vi "Dashboard Main.vi"() -> ()   [LabVIEW 2013]
uses:
  <vilib>/Rock Robotics/WPI/Camera/WPI_CameraExposure Priority Values.ctl
  <vilib>/Rock Robotics/WPI/Camera/WPI_CameraWhite Balance Values.ctl
  <vilib>/Rock Robotics/WPI/Camera/WPI_CameraExposure Values.ctl
  <vilib>/Rock Robotics/WPI/Camera/WPI_CameraImageSize.ctl
  <vilib>/vision/Image Controls.llb/IMAQ Image.ctl
  <vilib>/Utility/error.llb/DialogType.ctl
  <vilib>/Utility/file.llb/Write To Spreadsheet File (string).vi
  <vilib>/addons/control/pid/pid.llb/PID Control Input Filter (DBL).vi
  <vilib>/vision/NI_Vision_Development_Module.lvlib
  <vilib>/addons/control/pid/NI_PID_pid.lvlib
  <vilib>/Analysis/NI_AALBase.lvlib
panel:
  in  "Cam File":enum32{"Auto Detect", "Sting", "Sister-Sting"}(radio)
  out "Person Change":bool
  out "standard deviation":dbl(knob) scale=0.0..1.0
  out "compass lag":dbl
  out "Frame Number":i32
  in  "Bank Shot":bool
  out "Status":T1(ring)
  out "Mode":enum8{"Tele-Op", "Auto", ""}(ring)=enum.""
  out "Ang":dbl(knob) scale=-10.0..10.0
  out "Dist":dbl(knob) scale=12.0..32.0
  out "Ball Count":dbl
  out "RIO Fire":bool
  in  "TargetMarginMin":dbl=5.0
  in  "TargetMarginMax":dbl=5.0
  in  "SteadyTimeLimit":dbl=1.0
  out "Processed Image 2":T2(plugin-control)
  out "Purple Settings":T3
  out "Red Settings":T3
  out "Blue Settings":T3
  out "Lum Range":cluster{i32, i32}
  out "Sat Range":cluster{i32, i32}
  out "Hue Range":cluster{i32, i32}
  out "SubFrame2":i32
  out "SubFrame1":i32
  out "Left Target Valid":bool
  out "Y2":dbl
  out "Right Target Valid":bool
  out "ScoreLowerLimitsA":dbl[](array[numeric])
  out "Processed Image Source":T2
  out "Scored Particle Info":T4(array[cluster])
  out "Scored Particle Info 2":T4(array[cluster])
  out "Processed Image 2 Source":T2
  out "Raw Image Out 2":T2
  out "Raw Image Out":T2
  out "Processed Image":T2(plugin-control)
  out "Right Target":T5
  out "Left Target":T5
  out "TargetAcquired":bool
  out "Rotated Image 2":T2(plugin-control)
  out "Rotated Image":T2(plugin-control)
  out "Softstops!":bool caption="FAILSAFE!"
  in  "Tab Control":T6(tab)
  out "Turrett SLOW Mode":bool
  out "Collector System Enabled":bool
  out "Shooter RPM":cluster{dbl, dbl}(knob)={0.0, 3890.9503656333954} scale=0.0..4000.0
  out "Limit Right":bool
  out "Limit Left":bool
  out "Turret Postition":cluster{dbl, dbl}(knob)={0.0, 3.981103692185485} scale=-240.0..60.0
  out "Home":bool
  out "1":bool
  out "2":bool
  out "3":bool
  out "Bridge Balance":bool
  out "Intake Direction":bool
  out "High Gear":bool
  out "Low Gear":bool
  out "Battery Voltage":dbl(slide) scale=8.0..14.0
  out "Distance From Target":dbl
  out "Angle to Target":dbl
  out "Entrance":bool
  out "Lower Belt":bool
  out "Upper Belt":bool
  out "Primed":bool
  out "AngleTolerance":dbl
  out "Auto Targeting":bool
  out "In Angle Range":bool
  out "Turret Enc":dbl
  out "Compass":dbl(knob) scale=0.0..-180.0
  out "Shooter Ready":bool
  out "Right Drive":dbl
  out "Left Drive":dbl
  out "Gyro":dbl(knob) scale=-180.0..180.0
  out "Robot IP Address":string
  out "In Angle?":bool
  out "Personality":string
  out "Cam File":string
  out "Lag":bool
  in  "Score Lower Limits":T7={"Rect Coverage"=76.0, "Aspect Ratio"=100.0, "X Edge Strength"=40.0, "Y Edge Strength"=60.0}
  in  "Aspect Ratio Upper":dbl=200.0
  in  "Distance Change":dbl
  in  "Left FOV":dbl=35.0
  in  "Right FOV":dbl=35.0
  in  "Area Size Limit":i32=444
  in  "Particle Count Limit":i32=8
  in  "Shift Right Camera  Right (Pixels)":dbl=-23.0
  in  "Shift Left Camera Right (Pixels)":dbl
  in  "Camera Width":dbl=18.0
  in  "Distance M Correction":dbl=1.3463
  in  "Distance B \nCorrection":dbl=2.0300000000000002
  out "Target Data":T8
  out "FPS":dbl
  in  "Angle Correction":dbl=1.0
  out "X1":dbl
  out "Y1":dbl
  out "X2":dbl
  in  "Color Level":i32(slide)=50 min=0 max=100 scale=0.0..100.0
  in  "Sharpness":i32(slide) min=0 max=100 scale=0.0..100.0
  in  "Brightness":i32(slide)=50 min=0 max=100 scale=0.0..100.0
  in  "Camera Settings":T10={"fps"=30, "compression"=30, "Image Size"=enum."640x480"}
  in  "Exposure Priority":T11=enum."Prioritize frame rate"
  in  "Exposure":T12=enum."Flicker-free 60 Hz"
  in  "White Balance":T13=enum."Fixed fluorescent 1"
  in  "Processed":bool
  in  "Sat":i32=255
  in  "Lum":i32=255
  in  "Hue":i32=40
  in  "Hue":i32(knob)=206 scale=0.0..255.0
  in  "Saturation":i32=80
  in  "Luminance":i32=20
  in  "LED Colors":enum16{"Blue", "Red", "Purple", "Test"}(ring)=enum."Purple"
  in  "Reload":bool
  in  "Write Blue":bool
  in  "Write Red":bool
  in  "Write Purple":bool
  in  "Calibrate Cameras":bool
  in  "Distance to Target":dbl=16.8
  out "FIRE!":bool
  out "Dashboard Datatype Warning":string="Warning: The Dashboard Datatype used by the robot project and this dashboard do not match.\nSee diagram for more details."
  # "The different autonomous can be set up from the driver station. Set up as binary.\n1 (001) - Default\n2 (010)- Coopertition (have another bot feed us balls that we can shoot, untested)\n3 (011)- X second delay to shooting first ball (NO BRIDGE)\n4 (100) - X second delay to shooting first ball (Go for bridge)\n5 (101)- Reverse Order (Puts down bridge then shoots, untested)"
  # "Ball Count"
  # "Communications"
  # "Margin"
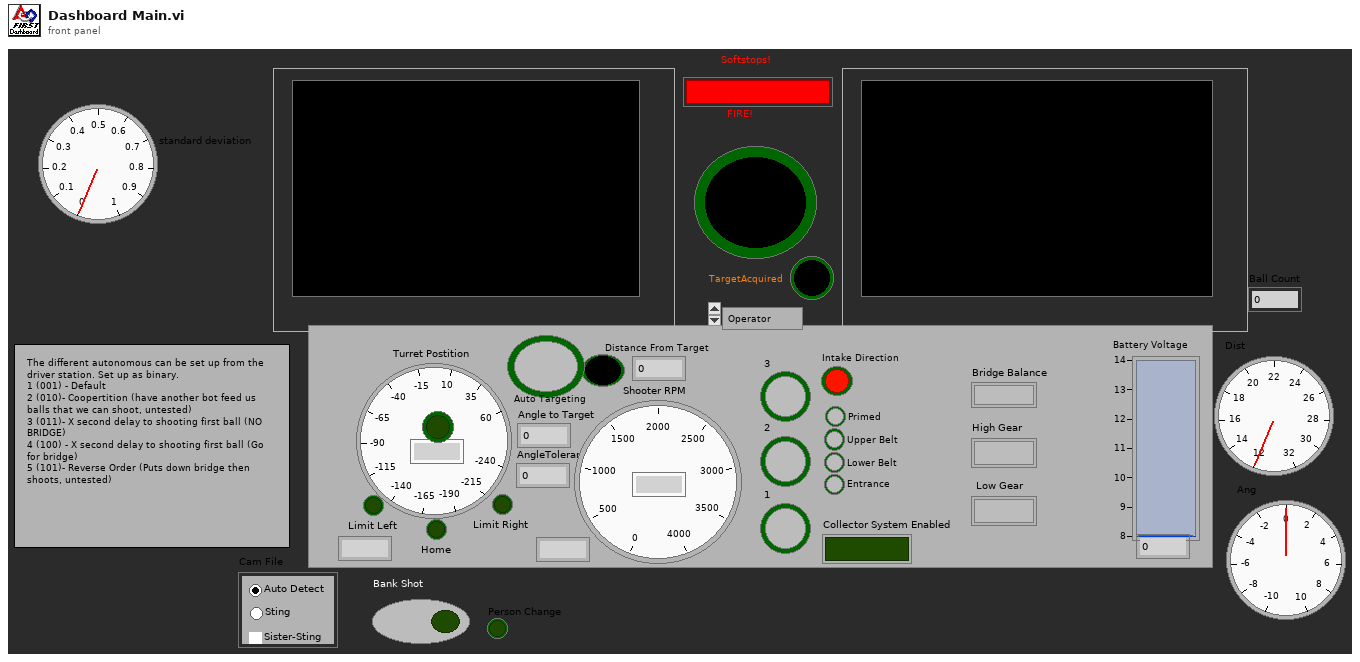
[diagram p1: front panel]
types:
  T1 = enum8{"Disconnected", "E-Stop", "Disabled", "Enabled"}
  T2 = typedef "IMAQ Image.ctl" = refnum<image>
  T3 = cluster{cluster{"Hue":i32, "Sat":i32, "Lum":i32}, cluster{"HueM":i32, "SatM":i32, "LumM":i32}}
  T4 = cluster{cluster{"Left":dbl, "Top":dbl, "Right":dbl, "Bottom":dbl}, dbl[]}[]
  T5 = cluster{"Left":dbl, "Top":dbl, "Right":dbl, "Bottom":dbl}
  T6 = enum32{"Operator", "Diagnotics", "Vision", "Camera Conf"}
  T7 = cluster{"Rect Coverage":dbl, "Aspect Ratio":dbl, "X Edge Strength":dbl, "Y Edge Strength":dbl}
  T8 = cluster{i32, dbl, "Angle to Target":dbl, "Valid Target":bool}
  T9 = typedef "WPI_CameraImageSize.ctl" = enum16{"640x480", "320x240", "160x120"}
  T10 = cluster{"fps":i32, "compression":i32, "Image Size":T9}
  T11 = typedef "WPI_CameraExposure Priority Values.ctl" = enum16{"None", "Prioritize frame rate", "Prioritize image quality"}
  T12 = typedef "WPI_CameraExposure Values.ctl" = enum16{"Auto", "Flicker-free 50 Hz", "Flicker-free 60 Hz", "Hold current"}
  T13 = typedef "WPI_CameraWhite Balance Values.ctl" = enum16{"Auto", "Fixed indoor", "Fixed outdoor 1", "Fixed outdoor 2", "Fixed fluorescent 1", "Fixed fluorescent 2", "Hold current"}
  T14 = cluster{"Bridge Balance":bool, "Gyro":dbl, "Left Drive":dbl, "Right Drive":dbl, "Shooter Ready":bool, "Compass":dbl, "Turret Enc":dbl, "Gear":u16, "Turret Postion":dbl, "Turret Bump":bool, "Collector System Enabled?":bool, "Personality":string}
  T15 = cluster{"Ball Count":dbl, "Shooter RMP":dbl, "FIRE":bool, "FailSafe":bool, "Entrance":bool, "Lower Belt":bool, "Upper Belt":bool, "Primed":bool, "Intake":bool, "Right Limit":bool, "Home":bool, "Left Limit":bool, "Auto Target ?":bool}
  T16 = typedef "Image Type" = u32
  T17 = typedef "DialogType.ctl" = u16
  T18 = cluster{"Competition mode":bool, "Robot Link":bool, "Autonomous":bool, "Enabled":bool, "E-Stop":bool}
  T19 = cluster{"Distance From Target":dbl, "Distance From Target":dbl, "Distance From Target":dbl, "Distance From Target":dbl, "Distance From Target":dbl}
  T20 = cluster{"Shooter RMP":dbl, "Shooter RPM Control":dbl}
  T21 = typedef "WPI_CameraDevRef.ctl" = cluster{"Camera Address":string, "CameraStatus":errorcluster, "Acquire Image Notifier":refnum<notifier>}
  T22 = typedef "LVRectTypeDef.ctl" = cluster{"Left":i16, "Top":i16, "Right":i16, "Bottom":i16}
  T23 = cluster{"SteadyTime":dbl, "TargetMarMax":dbl, "TargetMarMin":dbl}
  T24 = cluster{cluster{"LFOV":dbl, "RFOV":dbl, "CamW":dbl}, cluster{"Ladj":dbl, "Radj":dbl, "Dadj":dbl}, cluster{"CamM":dbl, "CamB":dbl, "AngM":dbl}, "Color":u16}
  T25 = cluster{"Hue":i32, "Saturation":i32, "Luminance":i32}
  T26 = cluster{cluster{"Hue":i32, "Saturation":i32, "Luminance":i32}, cluster{"Hue":i32, "Sat":i32, "Lum":i32}}
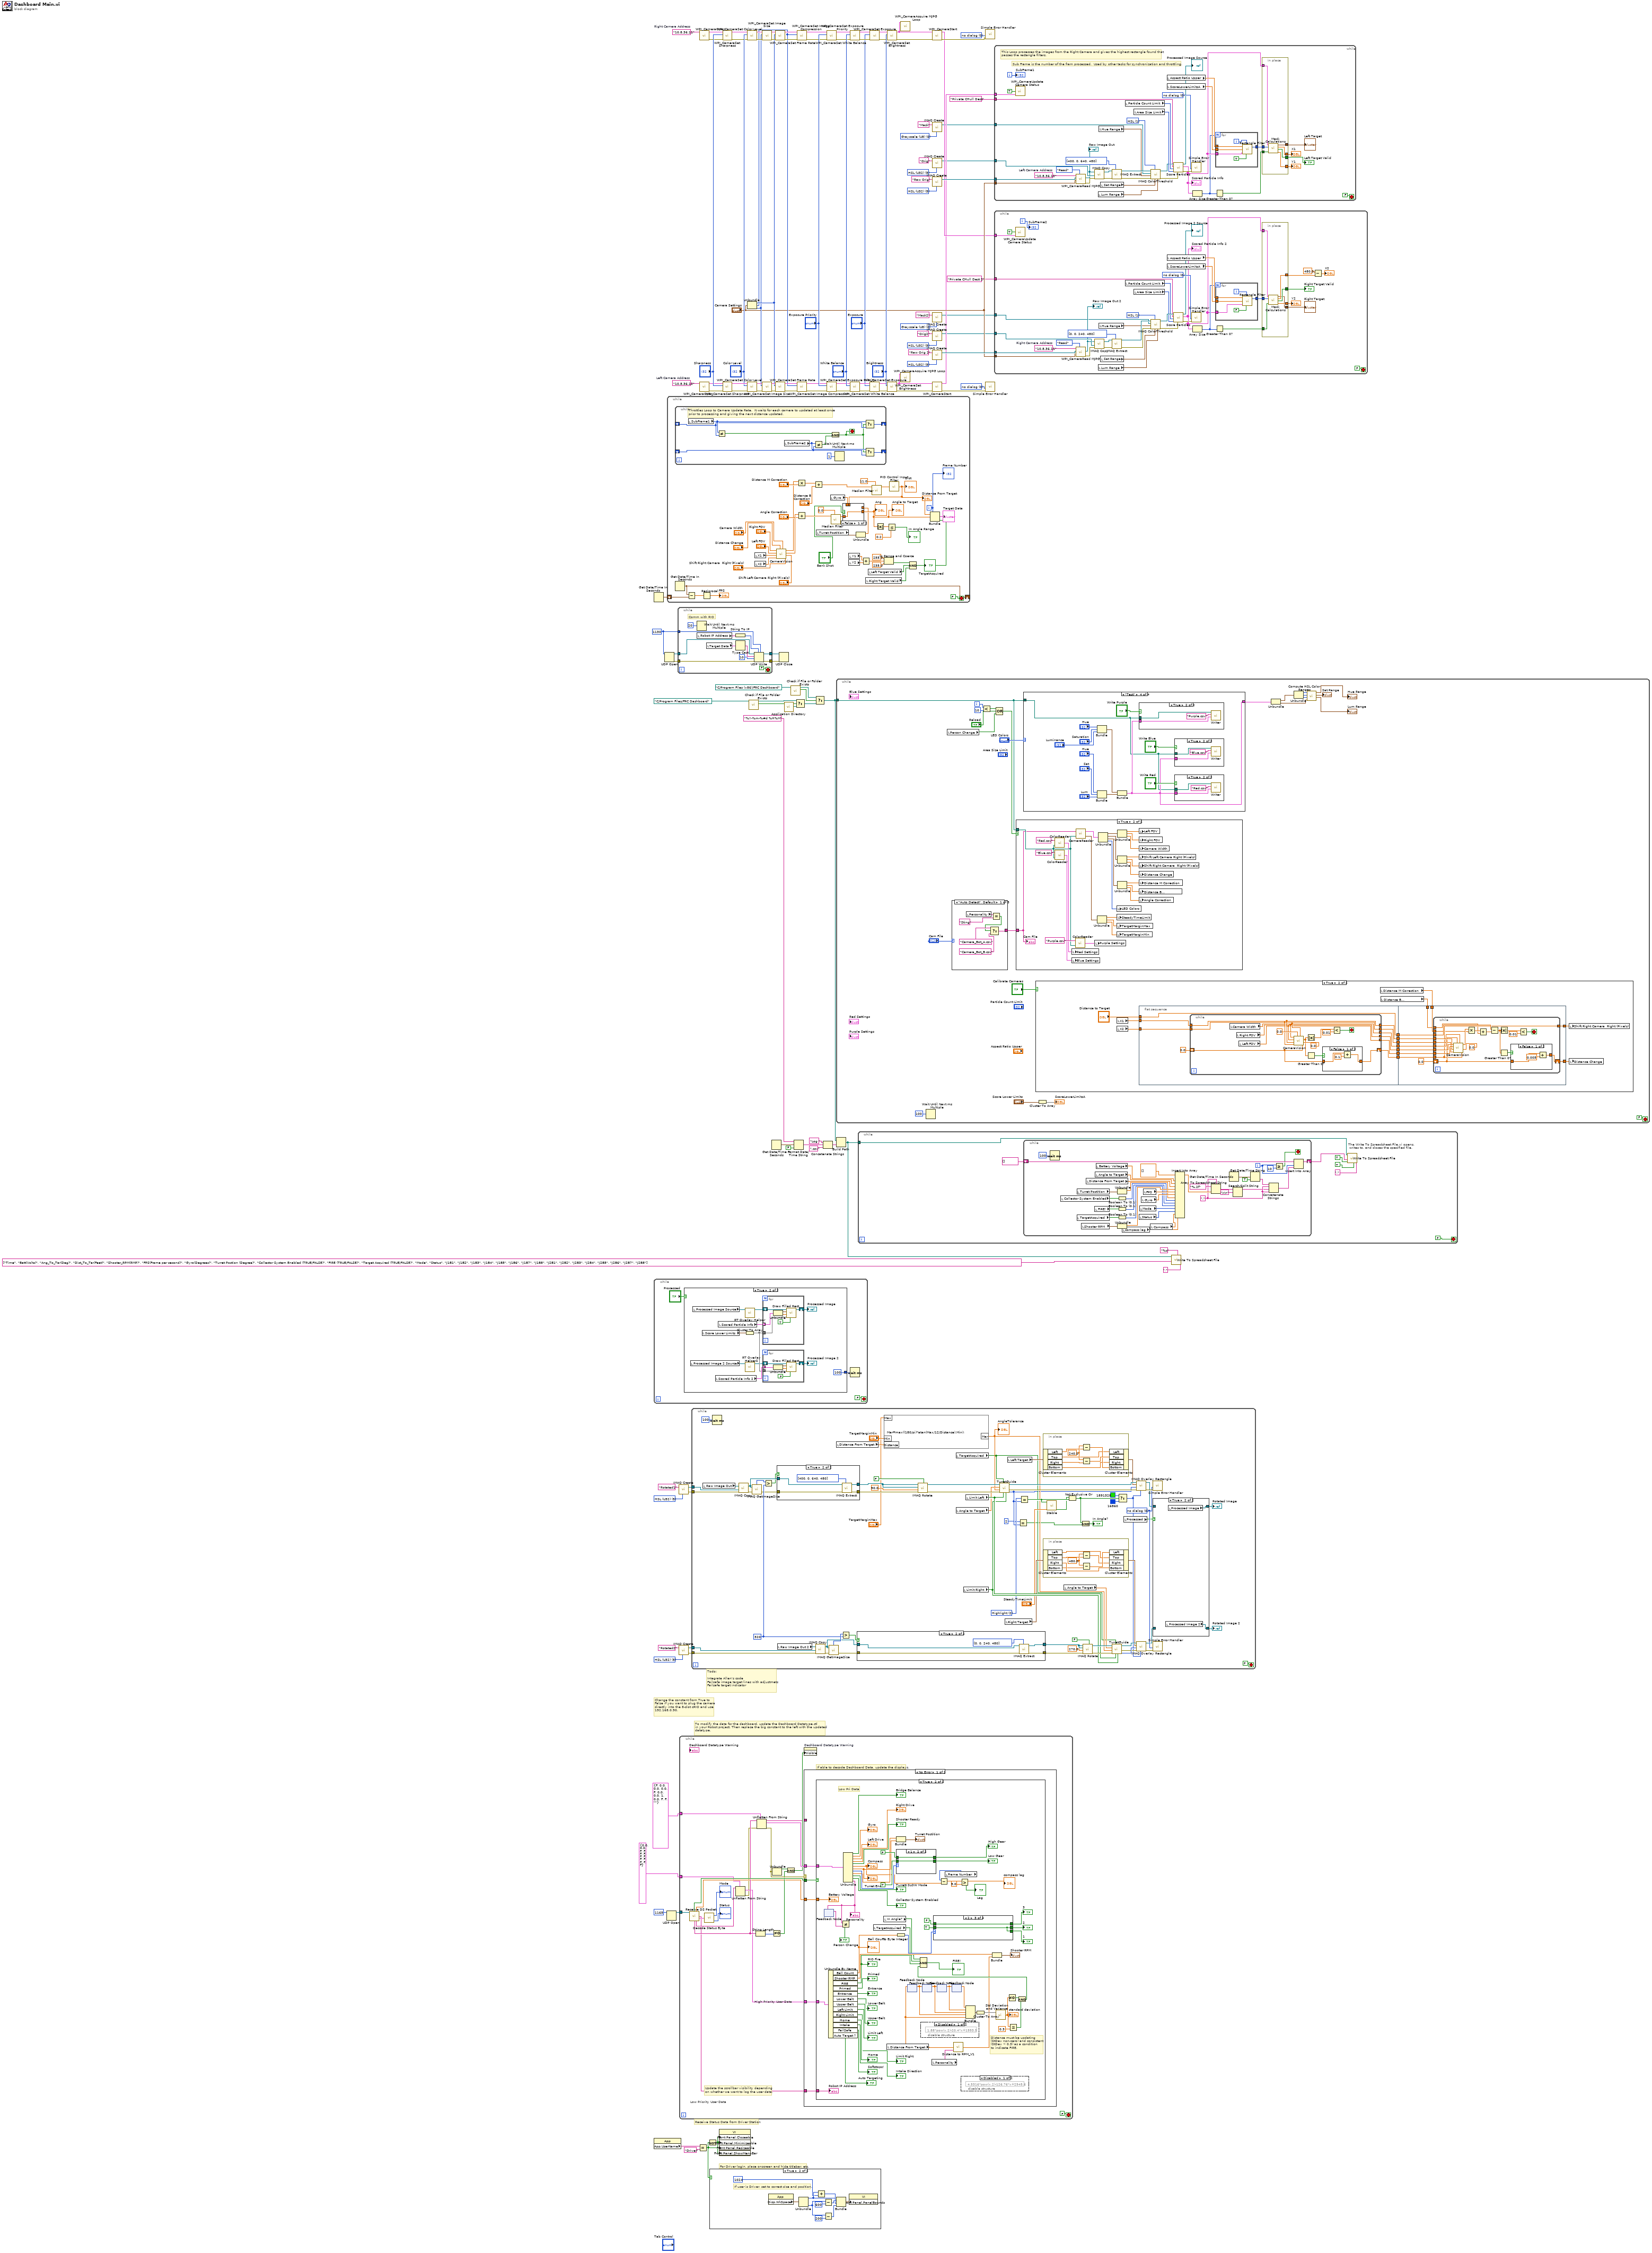
[diagram p0: block diagram]
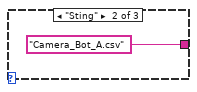
[diagram p2: hidden frame]
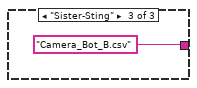
[diagram p3: hidden frame]
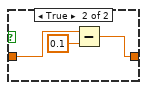
[diagram p5: hidden frame]
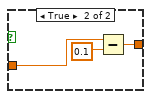
[diagram p6: hidden frame]
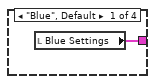
[diagram p8: hidden frame]
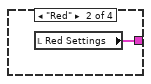
[diagram p9: hidden frame]
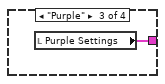
[diagram p10: hidden frame]
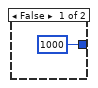
[diagram p14: hidden frame]
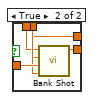
[diagram p19: hidden frame]
diagram:
  w7 = T16 5 items=["Grayscale (U8)", "Grayscale (I16)", "Grayscale (SGL)", "Complex (CSG)", "RGB (U32)", "HSL (U32)", "RGB (U64)", "Grayscale (U16)"] ("Image Type")
  w9 = T16 0 items=["Grayscale (U8)", "Grayscale (I16)", "Grayscale (SGL)", "Complex (CSG)", "RGB (U32)", "HSL (U32)", "RGB (U64)", "Grayscale (U16)"] ("Image Type")
  w12 = T16 0 items=["Grayscale (U8)", "Grayscale (I16)", "Grayscale (SGL)", "Complex (CSG)", "RGB (U32)", "HSL (U32)", "RGB (U64)", "Grayscale (U16)"] ("Image Type")
  w16 = T16 5 items=["Grayscale (U8)", "Grayscale (I16)", "Grayscale (SGL)", "Complex (CSG)", "RGB (U32)", "HSL (U32)", "RGB (U64)", "Grayscale (U16)"] ("Image Type")
  w21 = T17 0 items=["no dialog", "OK message", "continue or stop message", "OK message + warnings", "continue/stop + warnings"] ("type of dialog (OK msg:1)")
  w22 = T17 0 items=["no dialog", "OK message", "continue or stop message", "OK message + warnings", "continue/stop + warnings"] ("type of dialog (OK msg:1)")
  w28 = T16 5 items=["Grayscale (U8)", "Grayscale (I16)", "Grayscale (SGL)", "Complex (CSG)", "RGB (U32)", "HSL (U32)", "RGB (U64)", "Grayscale (U16)"] ("Image Type")
  w30 = T16 5 items=["Grayscale (U8)", "Grayscale (I16)", "Grayscale (SGL)", "Complex (CSG)", "RGB (U32)", "HSL (U32)", "RGB (U64)", "Grayscale (U16)"] ("Image Type")
  w26 = "10.8.36.11"  # Right Camera Address
  w32 = "10.8.36.12"  # Left Camera Address
  w107 = T16 5 items=["Grayscale (U8)", "Grayscale (I16)", "Grayscale (SGL)", "Complex (CSG)", "RGB (U32)", "HSL (U32)", "RGB (U64)", "Grayscale (U16)"] ("Image Type")
  w110 = T16 5 items=["Grayscale (U8)", "Grayscale (I16)", "Grayscale (SGL)", "Complex (CSG)", "RGB (U32)", "HSL (U32)", "RGB (U64)", "Grayscale (U16)"] ("Image Type")
  w111 = u16 1130 ("port")
  # "Todo: \n\nIntegrate Allen's code\nFailsafe image target lines with adjustmets\nFailsafe target indicator"
  # "Change the constant from True to\nFalse if you want to plug the camera\ndirectly into the 8-slot cRIO and use\n192.168.0.90."
  # "For Driver login, place onscreen and hide titlebar, etc."
  # "To modify the data for the dashboard, update the Dashboard Datatype.ctl\nin your Robot project. Then replace the big constant to the left with the updated\ndatatype."
  # "Receive Status Data from Driver Station"
  n1 = Get Date/Time In Seconds() -> (seconds since 1Jan1904=w116:timestamp)
  n2 = while {
    stop <- FALSE stop-if-true
    n3 = case shown="True" "Processed" {
      tunnel: [u32 1000 ("milliseconds to wait") u32 100 ("milliseconds to wait")] -> w121
      frame False {
      }
      frame True {
        n4 = local read "Processed Image 2 Source"() -> (w134:T2)
        n5 = local read "Processed Image Source"() -> (w131:T2)
        n6 = local read "Score Lower Limits"() -> (w135:T7)
        n7 = local read "Scored Particle Info 2"() -> (w133:T4)
        n8 = local read "Scored Particle Info"() -> (w130:T4)
        n9 = call "RT Overlay Helper.vi"("Refnum in"=w131) -> ("Refnum out"=w126:T2)  [unwired: 10 in]
        n10 = Cluster To Array(cluster=w135) -> (array=w132:dbl[])
        n11 = call "RT Overlay Helper2.vi"("Refnum in"=w134) -> ("Refnum out"=w128:T2)  [unwired: 10 in]
        n12 = for {
          shift-right: [w141] -> w127
          shift-left: w126 -> [w142]
          tunnel: w130 -> [w138] mode=indexing
          tunnel: w132 -> [w137]
          n13 = Unbundle(w138) -> (w139:T5, w140:dbl[])
          n14 = call "Draw Filled Rect.vi"("Left"=TRUE, "Limits"=w137, "Scores"=w140, "Bounding Box"=w139, "image in"=w142) -> ("image out"=w141:T2)  [unwired: 6 in]
        }
        "Processed Image" <- w127
        n15 = for {
          shift-right: [w148] -> w129
          shift-left: w128 -> [w149]
          tunnel: w133 -> [w145] mode=indexing
          tunnel: w132 -> [w144]
          n16 = Unbundle(w145) -> (w146:T5, w147:dbl[])
          n17 = call "Draw Filled Rect.vi"("Left"=FALSE, "Limits"=w144, "Scores"=w147, "Bounding Box"=w146, "image in"=w149) -> ("image out"=w148:T2)  [unwired: 6 in]
        }
        "Processed Image 2" <- w129
      }
    }
    n18 = Wait (ms)(milliseconds to wait=w121) -> ()  [unwired: 1 out]
  }
  n19 = property class="App"() -> ("App.UserName"=w117:string)  [unwired: 2 in, 2 out]
  n20 = UDP Open(11:w111) -> (port=w114:refnum<k16>, 0:w112:errorcluster)  [unwired: 4 in, 1 out]
  n21 = UDP Open(11:u16 1165 ("port")) -> (port=w119:refnum<k16>)  [unwired: 2 in, 4 out]
  n22 = while {
    shift-right: [w168] -> _
    shift-left: w116 -> [w190]
    i -> [w182]
    stop <- FALSE stop-if-true
    n23 = while {
      shift-right: [w209] -> _
      shift-left: _ -> [w207]
      shift-right: [w206] -> _
      shift-left: _ -> [w205]
      stop <- w201 stop-if-true
      # "Throttles Loop to Camera Update Rate.  It waits for each camera to updated at least once\nprior to processing and giving the next distance updated."
      n24 = local read "SubFrame1"() -> (w208:i32)
      n25 = Not Equal?(x=w208, y=w207) -> (x != y?=w202:bool)
      n26 = local read "SubFrame2"() -> (w204:i32)
      n27 = Not Equal?(x=w204, y=w205) -> (x != y?=w203:bool)
      n28 = And(x=w202, y=w203) -> (x .and. y?=w201:bool)
      n29 = Wait Until Next ms Multiple(millisecond multiple=u32 1) -> ()  [unwired: 1 out]
      n30 = Select(t=w208, s=w201, f=w207) -> (s? t:f=w209:i32)
      n31 = Select(t=w204, s=w201, f=w205) -> (s? t:f=w206:i32)
    }
    n32 = Get Date/Time In Seconds() -> (seconds since 1Jan1904=w168:timestamp)
    n33 = Subtract(x=w168, y=w190) -> (x-y=w165:dbl)
    n34 = Reciprocal(x=w165) -> (1/x=→"FPS":dbl)
    n35 = local read "X1"() -> (w170:dbl)
    n36 = local read "X2"() -> (w174:dbl)
    n37 = call "CameraVision.vi"("X2 Change"="Shift Right Camera  Right (Pixels)", "X1 Change"="Shift Left Camera Right (Pixels)", "W"="Camera Width", "Distance Change"="Distance Change", "x2"=w174, "x"=w170, "Left FOV"="Left FOV", "Right FOV"="Right FOV") -> ("Angle to Target"=w184:dbl, "Distance to Target"=w181:dbl)  [unwired: 1 in]
    n38 = Multiply(x=w181, y="Distance M Correction") -> (x*y=w176:dbl)
    n39 = Add(x=w184, y="Angle Correction") -> (x+y=w163:dbl)
    n40 = Add(x=w176, y="Distance B \nCorrection") -> (x+y=w162:dbl)
    n41 = local read "Turret Postition"() -> (w154:cluster{dbl, dbl})
    n42 = local read "Gyro"() -> (w152:dbl)
    n43 = call "Median Filter.vi"("Initial Value"=0.0, "Variable"=w163) -> ("Filtered Value"=w156:dbl)  [unwired: 9 in]
    n44 = local read "Y1"() -> (w169:dbl)
    n45 = local read "Y2"() -> (w172:dbl)
    n46 = Unbundle(w154) -> (w153:dbl)  [unwired: 1 out]
    n47 = Add(x=w169, y=w172) -> (x+y=w179:dbl)
    n48 = local read "Right Target Valid"() -> (w173:bool)
    n49 = local read "Left Target Valid"() -> (w171:bool)
    n50 = call "Median Filter.vi"("Initial Value"=11.0, "Variable"=w162) -> ("Filtered Value"=w161:dbl)  [unwired: 9 in]
    n51 = In Range and Coerce(upper limit=255.0, x=w179, lower limit=235.0) -> (In Range?=w150:bool)  [unwired: 1 out]
    n52 = call-poly <vilib>:"PID Control Input Filter.vi"("input"=w161) -> ("output"=w155:dbl)  [unwired: 4 in]
    "Distance From Target" <- w155
    "Dist" <- w155
    n53 = case shown="False" "Bank Shot" {
      tunnel: [w195 w200] -> w157
      tunnel: w156 -> [w195 w199]
      tunnel: w155 -> [_ w198]
      tunnel: w153 -> [_ w197]
      tunnel: w152 -> [_ w196]
      frame False {
      }
      frame True {
        n54 = call "Bank Shot.vi"("L (ft)"=w198, "Camera (deg)"=w199, "Turret (deg)"=w197, "Gryo (deg)"=w196) -> ("C Prime"=w200:dbl)  [unwired: 6 in, 1 out]
      }
    }
    "Angle to Target" <- w157
    "Ang" <- w157
    n55 = Absolute Value(x=w157) -> (abs(x)=w160:dbl)
    n56 = Less Or Equal?(x=w160, y=0.2) -> (x <= y?=→"In Angle Range":bool)
    n57 = Compound Arithmetic op=AND(w150, w171, w173) -> (w175:bool)
    "TargetAcquired" <- w175
    n58 = Bundle(w182, "output"=w155, "C Prime"=w157, w175) -> (→"Target Data":cluster{i32, "output":dbl, "C Prime":dbl, bool})  [unwired: 1 in]
    "Frame Number" <- w182
  }
  n59 = while {
    tunnel: [w217] -> w115
    tunnel: w114 -> [w216]
    tunnel: [w218] -> w113
    tunnel: w112 -> [w213]
    tunnel: w111 -> [w212]
    stop <- FALSE stop-if-true
    # "Comm with RIO"
    n60 = Wait Until Next ms Multiple(millisecond multiple=u32 20) -> ()  [unwired: 1 out]
    n61 = local read "Robot IP Address"() -> (w211:string)
    n62 = local read "Target Data"() -> (w219:T8)
    n63 = String To IP(1:w211) -> (0:w220:u32)
    n64 = Type Cast(x=w219) -> (*(type *) &x=w215:string)  [unwired: 1 in]
    n65 = UDP Write(address=w220, port or service name=w212, connection ID=w216, data in=w215, 8:w213, 9:10 ("timeout ms (25000)")) -> (error out=w218:errorcluster, 3:w217:refnum<k16>)
  }
  n66 = call "IMAQ Create"("Image Name"="Rotated1", "Image Type"=w110) -> ("New Image"=w106:T2, "error out"=w103:errorcluster)  [unwired: 2 in, 1 out]
  n67 = call "IMAQ Create"("Image Name"="Rotated2", "Image Type"=w107) -> ("New Image"=w105:T2, "error out"=w104:errorcluster)  [unwired: 2 in, 1 out]
  n68 = while {
    tunnel: w119 -> [w241]
    tunnel: T14 {"Bridge Balance"=FALSE, "Gyro"=0.0, "Left Drive"=0.0, "Right Drive"=0.0, "Shooter Ready"=FALSE, "Compass"=0.0, "Turret Enc"=0.0, "Gear"=1, "Turret Postion"=0.0, "Turret Bump"=FALSE, "Collector System Enabled?"=FALSE, "Personality"=""} ("Dashboard Data") -> [w240]
    tunnel: T15 {"Ball Count"=0.0, "Shooter RMP"=0.0, "FIRE"=FALSE, "FailSafe"=FALSE, "Entrance"=FALSE, "Lower Belt"=FALSE, "Upper Belt"=FALSE, "Primed"=FALSE, "Intake"=FALSE, "Right Limit"=FALSE, "Home"=FALSE, "Left Limit"=FALSE, "Auto Target ?"=FALSE} ("HiPri") -> [w227]
    stop <- FALSE stop-if-true
    # "High Priority User Data"
    # "Low Priority User Data"
    # "Update the scrollbar visibility depending\non whether we want to log the user data."
    # "If able to decode Dashboard Data, update the displays."
    n69 = call "Receive DS Packet.vi"("Recv Socket"=w241) -> ("New Dashboard Data"=w237:bool, "Battery"=w229:sgl, "Robot IP Address"=w228:string, "Status"=w242:T18, "Low Priority User Data"=w231:string, "High Priority User Data"=w230:string)  [unwired: 1 in, 8 out]
    n70 = call "Decode Status Byte.vi"("Status Byte"=w242) -> ("Mode"=→"Mode":enum8{"Tele-Op", "Auto", ""}, "Status"=→"Status":T1)
    n71 = Unflatten From String(type=w227, binary string=w230) -> (value=w226:T15, error out=w225:errorcluster)  [unwired: 1 in, 3 out]
    n72 = String Length(string=w231) -> (length=w232:i32)
    n73 = Unflatten From String(type=w240, binary string=w231, error in (no error)=w225) -> (rest of the binary string=w233:string, value=w239:T14, error out=w238:errorcluster)  [unwired: 2 out]
    n74 = Not Equal To 0?(x=w232) -> (x != 0?=w235:bool)
    n75 = Unbundle(w238) -> ("status"=w234:bool)  [unwired: 2 out]
    n76 = And(x=w234, y=w235) -> (x .and. y?=w236:bool)
    n77 = property on="Dashboard Datatype Warning" class="Str"("Visible"=w236) -> ()  [unwired: 2 in, 2 out]
    n78 = case shown="No Error" w238 {
      tunnel: w239 -> [w248 _]
      tunnel: w237 -> [w247 _]
      tunnel: w233 -> [_ _]
      tunnel: w229 -> [w246 _]
      tunnel: w228 -> [w245 _]
      tunnel: w226 -> [w244 _]
      frame No Error {
        n79 = case shown="True" w247 {
          tunnel: w248 -> [_ w312]
          tunnel: w246 -> [_ w311]
          tunnel: w245 -> [_ w310]
          tunnel: w244 -> [_ w309]
          frame False {
            # "Don't update if the robot hasn't sent new data"
          }
          frame True {
            # "Distance must be updating\n(StDev non-zero) and consistent\n(StDev < 0.3) as a condition\nto indicate FIRE."
            # "Low Pri Data"
            n80 = feedback #1() -> (w250:string)  [unwired: 1 in]
            n81 = Unbundle By Name(w309) -> ("Ball Count"=w273:dbl, "Shooter RMP"=w282:dbl, "FIRE"=w276:bool, "Primed"=→"Primed":bool, "Entrance"=→"Entrance":bool, "Lower Belt"=→"Lower Belt":bool, "Upper Belt"=→"Upper Belt":bool, "Left Limit"=→"Limit Left":bool, "Right Limit"=→"Limit Right":bool, "Home"=→"Home":bool, "Intake"=→"Intake Direction":bool, "FailSafe"=→"Softstops!":bool, "Auto Target ?"=→"Auto Targeting":bool)
            "RIO Fire" <- w276
            "Ball Count" <- w273
            n82 = Unbundle(w312) -> ("Bridge Balance"=→"Bridge Balance":bool, "Gyro"=→"Gyro":dbl, "Left Drive"=→"Left Drive":dbl, "Right Drive"=→"Right Drive":dbl, "Shooter Ready"=→"Shooter Ready":bool, "Compass"=w271:dbl, "Turret Enc"=w275:dbl, "Gear"=w308:u16, "Turret Postion"=w280:dbl, "Turret Bump"=→"Turrett SLOW Mode":bool, "Collector System Enabled?"=→"Collector System Enabled":bool, "Personality"=w251:string)
            "Compass" <- w271
            "Turret Enc" <- w275
            "Personality" <- w251
            n83 = feedback-in #1(w251) -> ()
            n84 = Not Equal?(x=w251, y=w250) -> (x != y?=→"Person Change":bool)
            n85 = local read "TargetAcquired"() -> (w274:bool)
            n86 = local read "In Angle?"() -> (w277:bool)
            n87 = local read "Distance From Target"() -> (w254:dbl)
            n88 = Bundle("Turret Postion"=w280, "Turret Enc"=w275) -> (→"Turret Postition":cluster{"Turret Postion":dbl, "Turret Enc":dbl})  [unwired: 1 in]
            n89 = case shown="1" w308 {
              tunnel: [w320 w322] -> w307
              tunnel: FALSE -> [w319 w322]
              tunnel: TRUE -> [w320 w321]
              tunnel: [w319 w321] -> w304
              frame 0, Default {
              }
              frame 1 {
              }
            }
            "Low Gear" <- w304
            "High Gear" <- w307
            n90 = To Byte Integer(number=w273) -> (8bit integer=w289:i8)
            n91 = feedback-in #2(w254) -> ()
            n92 = feedback #2() -> (w262:dbl)  [unwired: 1 in]
            n93 = disable-structure shown="Disabled" {
              frame Disabled {
                n94 = expression code="1.88*pow(x,2)-20.4*x+1993.5"() -> ()  [unwired: 1 in, 1 out]
              }
              frame Enabled {
              }
            }
            n95 = feedback #3() -> (w263:dbl)  [unwired: 1 in]
            n96 = feedback-in #3(w262) -> ()
            n97 = local read "Personality"() -> (w252:string)
            n98 = case shown="2" w289 {
              tunnel: [w313 w314 w316 w318] -> w288
              tunnel: [w313 w314 w317 w318] -> w287
              tunnel: [w313 w315 w317 w318] -> w286
              tunnel: FALSE -> [w313 w314 w316 _]
              tunnel: TRUE -> [_ w315 w317 w318]
              frame 0, Default {
              }
              frame 1 {
              }
              frame 2 {
              }
              frame 3 {
              }
            }
            "3" <- w288
            "2" <- w287
            "1" <- w286
            n99 = feedback #4() -> (w264:dbl)  [unwired: 1 in]
            n100 = feedback-in #4(w263) -> ()
            n101 = local read "Frame Number"() -> (w270:i32)
            n102 = Subtract(x=w270, y=w271) -> (x-y=w269:dbl)
            "compass lag" <- w269
            n103 = feedback #5() -> (w265:dbl)  [unwired: 1 in]
            n104 = feedback-in #5(w264) -> ()
            n105 = call "Distance to RPM_V1.vi"("Personality"=w252, "Target Distance"=w254) -> ("Shooter RPM Control"=w253:dbl)  [unwired: 3 in]
            n106 = Greater?(x=w269, y=5.0) -> (0:→"Lag":bool)
            n107 = disable-structure shown="Disabled" {
              frame Disabled {
                n108 = expression code="4.5316*pow(x,2)-126.76*x+2945.6"() -> ()  [unwired: 1 in, 1 out]
              }
              frame Enabled {
              }
            }
            n109 = Bundle("Distance From Target"=w265, "Distance From Target"=w264, "Distance From Target"=w263, "Distance From Target"=w262, "Distance From Target"=w254) -> (w261:T19)  [unwired: 1 in]
            n110 = Cluster To Array(cluster=w261) -> (array=w260:dbl[])
            n111 = Bundle("Shooter RMP"=w282, "Shooter RPM Control"=w253) -> (→"Shooter RPM":T20)  [unwired: 1 in]
            n112 = call <vilib>:"Std Deviation and Variance.vi"("X"=w260) -> ("standard deviation"=w258:dbl)  [unwired: 1 in, 2 out]
            "standard deviation" <- w258
            n113 = Not Equal To 0?(x=w258) -> (x != 0?=w257:bool)
            n114 = Less Or Equal?(x=w258, y=0.3) -> (x <= y?=w256:bool)
            n115 = And(x=w257, y=w256) -> (x .and. y?=w255:bool)
            n116 = Compound Arithmetic op=AND(w276, w277, w274, w255) -> (→"FIRE!":bool)
            "Battery Voltage" <- w311
            "Robot IP Address" <- w310
          }
        }
      }
      frame Error {
        # "Your datatypes don't match. The Dashboard Datatype.ctl in your Robot project\nand the big constant to the left of the loop need to match."
      }
    }
  }
  n117 = while {
    tunnel: w106 -> [w380]
    tunnel: w105 -> [w388]
    tunnel: w104 -> [w372]
    tunnel: w103 -> [w364]
    stop <- FALSE ("stop") stop-if-true
    w354 = u32 2 items=["Frame", "Fill", "Highlight"] ("Drawing Mode (Frame)")
    w360 = T17 0 items=["no dialog", "OK message", "continue or stop message", "OK message + warnings", "continue/stop + warnings"] ("type of dialog (OK msg:1)")
    w377 = 320 ("y")
    n118 = local read "Raw Image Out"() -> (w381:T2)
    n119 = Wait (ms)(milliseconds to wait=u32 100) -> ()  [unwired: 1 out]
    n120 = call "IMAQ Copy"("error in (no error)"=w364, "Image Dst"=w380, "Image Src"=w381) -> ("error out"=w365:errorcluster, "Image Dst Out"=w379:T2)  [unwired: 3 in]
    n121 = call "IMAQ GetImageSize"("Image"=w379, "error in (no error)"=w365) -> ("X Resolution"=w383:i32, "error out"=w366:errorcluster)  [unwired: 2 in, 1 out]
    n122 = Greater?(x=w383, y=w377) -> (0:w345:bool)
    n123 = case shown="True" w345 {
      tunnel: [w418 w423] -> w382
      tunnel: w379 -> [w418 w422]
      tunnel: w366 -> [w417 w421]
      tunnel: [w417 w420] -> w361
      frame False {
      }
      frame True {
        n124 = call "IMAQ Extract"("Optional Rectangle"=i32[] [400, 0, 640, 480], "error in (no error)"=w421, "Image Src"=w422) -> ("error out"=w420:errorcluster, "Image Dst Out"=w423:T2)  [unwired: 7 in]
      }
    }
    n125 = local read "Raw Image Out 2"() -> (w387:T2)
    n126 = call "IMAQ Copy"("error in (no error)"=w372, "Image Dst"=w388, "Image Src"=w387) -> ("error out"=w363:errorcluster, "Image Dst Out"=w375:T2)  [unwired: 3 in]
    n127 = call "IMAQ GetImageSize"("Image"=w375, "error in (no error)"=w363) -> ("X Resolution"=w378:i32, "error out"=w362:errorcluster)  [unwired: 2 in, 1 out]
    n128 = local read "Distance From Target"() -> (w331:dbl)
    n129 = Greater?(x=w378, y=w377) -> (0:w344:bool)
    n130 = case shown="True" w344 {
      tunnel: w375 -> [w411 w416]
      tunnel: [w411 w415] -> w376
      tunnel: w362 -> [w410 w414]
      tunnel: [w410 w413] -> w367
      frame False {
      }
      frame True {
        n131 = call "IMAQ Extract"("Optional Rectangle"=i32[] [0, 0, 240, 480] ("Optional Rectangle 2"), "error in (no error)"=w414, "Image Src"=w416) -> ("error out"=w413:errorcluster, "Image Dst Out"=w415:T2)  [unwired: 7 in]
      }
    }
    n132 = formula code="Mar=max((180/pi)*atan(Max/12/Distance),Min);"("Max"="TargetMarginMax", "Min"="TargetMarginMin", "Distance"=w331) -> ("Mar"=w329:dbl)
    "AngleTolerance" <- w329
    n133 = call "IMAQ Rotate"("Maintain Size"=FALSE, "error in (no error)"=w361, "Angle (degrees)"=sgl 90.0, "Image Dst"=w382, "Image Src"=w382) -> ("error out"=w369:errorcluster, "Image Dst Out"=w374:T2)  [unwired: 5 in]
    n134 = local read "TargetAcquired"() -> (w328:bool)
    n135 = local read "Angle to Target"() -> (w356:dbl)
    n136 = local read "Limit Right"() -> (w358:bool)
    n137 = local read "Limit Left"() -> (w359:bool)
    n138 = call "TurretGuide.vi"("Right Stop"=w358, "Left Stop"=w359, "Angle Not Stale"=w328, "error in (no error)"=w369, "Angle Margin"=w329, "Angle to Target"=w356, "Image"=w374) -> ("Drawing Mode (Frame)"=w327:u32, "error out"=w355:errorcluster, "Image Out"=w357:T2)  [unwired: 2 in]
    n139 = local read "Right Target"() -> (w349:T5)
    n140 = local read "Left Target"() -> (w347:T5)
    n141 = Equal?(x=u32 2, y=w327) -> (x = y?=w323:bool)
    n142 = Equal?(x=w354, y=w327) -> (x = y?=w335:bool)
    n143 = in-place {
      w402 = 240.0 ("x")
      n144 = in-place-cluster #6(w347) -> ("Left"=w399:dbl, "Top"=w398:dbl, "Right"=w397:dbl, "Bottom"=w396:dbl)
      n145 = Subtract(x=w402, y=w399) -> (x-y=w400:dbl)
      n146 = Subtract(x=w402, y=w397) -> (x-y=w401:dbl)
      n147 = in-place-cluster #6("Left"=w398, "Top"=w401, "Right"=w396, "Bottom"=w400) -> (w346:T5)
    }
    n148 = in-place {
      w409 = 480.0 ("x")
      n149 = in-place-cluster #7(w349) -> ("Left"=w406:dbl, "Top"=w408:dbl, "Right"=w404:dbl, "Bottom"=w403:dbl)
      n150 = Subtract(x=w409, y=w408) -> (x-y=w405:dbl)
      n151 = Subtract(x=w409, y=w403) -> (x-y=w407:dbl)
      n152 = in-place-cluster #7("Left"=w407, "Top"=w406, "Right"=w405, "Bottom"=w404) -> (w348:T5)
    }
    n153 = call "Stable.vi"("Pulse Width (sec)"="SteadyTimeLimit", "Signal Input"=w335) -> ("Stable"=w334:bool)  [unwired: 9 in]
    n154 = local read "Angle to Target"() -> (w352:dbl)
    n155 = Not Exclusive Or(1:w335, 2:w334) -> (0:w324:bool)
    n156 = And(x=w324, y=w323) -> (x .and. y?=→"In Angle?":bool)
    n157 = call "IMAQ Rotate"("Maintain Size"=FALSE, "error in (no error)"=w367, "Angle (degrees)"=sgl 270.0, "Image Dst"=w376, "Image Src"=w376) -> ("error out"=w368:errorcluster, "Image Dst Out"=w373:T2)  [unwired: 5 in]
    n158 = call "TurretGuide.vi"("Right Stop"=w358, "Left Stop"=w359, "Angle Not Stale"=w328, "error in (no error)"=w368, "Angle Margin"=w329, "Angle to Target"=w352, "Image"=w373) -> ("Drawing Mode (Frame)"=w351:u32, "error out"=w350:errorcluster, "Image Out"=w353:T2)  [unwired: 2 in]
    n159 = Select(t=u32 1891328 ("Color"), s=w324, f=u32 16860 ("Color")) -> (s? t:f=w336:u32)
    n160 = local read "Processed"() -> (w339:bool)
    n161 = call "IMAQ Overlay Rectangle"("Color"=w336, "error in (no error)"=w355, "Drawing Mode (Frame)"=w327, "Rectangle"=w346, "Image"=w357) -> ("error out"=w370:errorcluster, "Image Out"=w343:T2)  [unwired: 1 in, 4 out]
    n162 = call "IMAQ Overlay Rectangle"("Color"=w336, "error in (no error)"=w350, "Drawing Mode (Frame)"=w351, "Rectangle"=w348, "Image"=w353) -> ("error out"=w371:errorcluster, "Image Out"=w340:T2)  [unwired: 1 in, 4 out]
    n163 = call <vilib>:"Simple Error Handler.vi"("type of dialog (OK msg:1)"=w360, "error in (no error)"=w370) -> ()  [unwired: 3 in, 5 out]
    n164 = case shown="True" w339 {
      tunnel: w343 -> [w393 _]
      tunnel: [w393 w395] -> w342
      tunnel: [w392 w394] -> w341
      tunnel: w340 -> [w392 _]
      frame False {
      }
      frame True {
        n165 = local read "Processed Image 2"() -> (w394:T2)
        n166 = local read "Processed Image"() -> (w395:T2)
      }
    }
    "Rotated Image 2" <- w341
    "Rotated Image" <- w342
    n167 = call <vilib>:"Simple Error Handler.vi"("type of dialog (OK msg:1)"=w360, "error in (no error)"=w371) -> ()  [unwired: 3 in, 5 out]
  }
  n168 = Equal?(x=w117, y="Driver") -> (x = y?=w102:bool)
  n169 = call <vilib>:"WPI_CameraOpen.vi"("Camera Address"=w26) -> ("error out"=w60:errorcluster, "CameraDevRef"=w64:T21)  [unwired: 2 in, 7 out]
  n170 = call <vilib>:"WPI_CameraOpen.vi"("Camera Address"=w32) -> ("error out"=w62:errorcluster, "CameraDevRef"=w63:T21)  [unwired: 2 in, 7 out]
  n171 = Not(x=w102) -> (.not. x?=w101:bool)
  n172 = case shown="True" w102 {
    frame False {
    }
    frame True {
      # "If user is Driver, set to correct size and position."
      n173 = property class="App"() -> ("Disp.WkSpace"=w433:T22)  [unwired: 2 in, 2 out]
      n174 = Unbundle(w433) -> ("Left"=w428:i16, "Bottom"=w424:i16)  [unwired: 2 out]
      n175 = Add(x=w428, y=1024) -> (x+y=w429:i32)
      n176 = Subtract(x=w424, y=600) -> (x-y=w430:i32)
      n177 = Subtract(x=w424, y=200) -> (x-y=w425:i32)
      n178 = Bundle("Left"=w428, w430, w429, w425) -> (w432:cluster{"Left":i16, i32, i32, i32})  [unwired: 1 out]
      n179 = property class="VI"("Front Panel.PanelBounds"=w432) -> ()  [unwired: 2 in, 2 out]
    }
  }
  n180 = property class="VI"("Front Panel.Closeable"=w101, "Front Panel.Minimizeable"=w101, "Front Panel.Resizeable"=w102, "Front Panel.ShowMenuBar"=w101) -> ()  [unwired: 2 in, 2 out]
  n181 = call <vilib>:"WPI_CameraSet Sharpness.vi"("error in (no error)"=w60, "Sharpness"="Sharpness", "CameraDevRef"=w64) -> ("error out"=w61:errorcluster, "CameraDevRef Out"=w73:T21)  [unwired: 7 in]
  n182 = call <vilib>:"WPI_CameraSet Sharpness.vi"("error in (no error)"=w62, "Sharpness"="Sharpness", "CameraDevRef"=w63) -> ("error out"=w78:errorcluster, "CameraDevRef Out"=w77:T21)  [unwired: 7 in]
  n183 = call <vilib>:"WPI_CameraSet Color Level.vi"("error in (no error)"=w61, "Color Level"="Color Level", "CameraDevRef"=w73) -> ("error out"=w39:errorcluster, "CameraDevRef Out"=w38:T21)  [unwired: 7 in]
  n184 = Unbundle("Camera Settings") -> ("fps"=w36:i32, "compression"=w35:i32, "Image Size"=w34:T9)
  n185 = call <vilib>:"WPI_CameraSet Color Level.vi"("error in (no error)"=w78, "Color Level"="Color Level", "CameraDevRef"=w77) -> ("error out"=w42:errorcluster, "CameraDevRef Out"=w43:T21)  [unwired: 7 in]
  n186 = call <vilib>:"Check if File or Folder Exists.vi"("path"=path "C:/Program Files/FRC Dashboard" ("file path (dialog if empty)")) -> ("file or folder exists?"=w96:bool, "dup path"=w98:path)  [unwired: 8 in, 1 out]
  n187 = call <vilib>:"WPI_CameraSet Image Size.vi"("error in (no error)"=w39, "Image Size"=w34, "CameraDevRef"=w38) -> ("error out"=w51:errorcluster, "CameraDevRef Out"=w50:T21)  [unwired: 7 in]
  n188 = call <vilib>:"WPI_CameraSet Image Size.vi"("error in (no error)"=w42, "Image Size"=w34, "CameraDevRef"=w43) -> ("error out"=w47:errorcluster, "CameraDevRef Out"=w46:T21)  [unwired: 7 in]
  n189 = Get Date/Time In Seconds() -> (seconds since 1Jan1904=w87:timestamp)
  n190 = call <vilib>:"WPI_CameraSet Frame Rate.vi"("error in (no error)"=w51, "Frame Rate (fps)"=w36, "CameraDevRef"=w50) -> ("error out"=w49:errorcluster, "CameraDevRef Out"=w48:T21)  [unwired: 7 in]
  n191 = call <vilib>:"WPI_CameraSet Frame Rate.vi"("error in (no error)"=w47, "Frame Rate (fps)"=w36, "CameraDevRef"=w46) -> ("error out"=w45:errorcluster, "CameraDevRef Out"=w44:T21)  [unwired: 7 in]
  n192 = UDP Close(connection ID=w115, 8:w113) -> ()  [unwired: 2 out]
  n193 = call <vilib>:"Application Directory.vi"() -> ("Application Directory"=w97:path)
  n194 = call <vilib>:"Check if File or Folder Exists.vi"("path"=path "C:/Program Files (x86)/FRC Dashboard" ("file path (dialog if empty)")) -> ("file or folder exists?"=w99:bool, "dup path"=w93:path)  [unwired: 8 in, 1 out]
  n195 = Format Date/Time String(time format string (%c)="%Y-%m-%#d %H%M", seconds (now)=w87, UTC format=FALSE ("want seconds? (F)")) -> (date/time string=w85:string)
  n196 = Select(t=w98, s=w96, f=w97) -> (s? t:f=w100:path)
  n197 = call <vilib>:"WPI_CameraSet Image Compression.vi"("error in (no error)"=w49, "Compression"=w35, "CameraDevRef"=w48) -> ("error out"=w37:errorcluster, "CameraDevRef Out"=w19:T21)  [unwired: 7 in]
  n198 = call <vilib>:"WPI_CameraSet Image Compression.vi"("error in (no error)"=w45, "Compression"=w35, "CameraDevRef"=w44) -> ("error out"=w40:errorcluster, "CameraDevRef Out"=w41:T21)  [unwired: 7 in]
  n199 = Select(t=w93, s=w99, f=w100) -> (s? t:f=w92:path)
  n200 = Concatenate Strings("Log " ("name or relative path"), w85, ".csv" ("name or relative path")) -> (w90:string)
  n201 = call <vilib>:"WPI_CameraSet Exposure Priority.vi"("error in (no error)"=w37, "Exposure Priority"="Exposure Priority", "CameraDevRef"=w19) -> ("error out"=w54:errorcluster, "CameraDevRef Out"=w55:T21)  [unwired: 7 in]
  n202 = call <vilib>:"WPI_CameraSet Exposure Priority.vi"("error in (no error)"=w40, "Exposure Priority"="Exposure Priority", "CameraDevRef"=w41) -> ("error out"=w52:errorcluster, "CameraDevRef Out"=w53:T21)  [unwired: 7 in]
  n203 = while {
    tunnel: w92 -> [w438]
    i -> [w441]
    stop <- FALSE stop-if-true
    n204 = Wait Until Next ms Multiple(millisecond multiple=u32 100) -> ()  [unwired: 1 out]
    n205 = local read "Person Change"() -> (w436:bool)
    n206 = case shown="\"Auto Detect\", Default" "Cam File" {
      tunnel: [w458 "Camera_Bot_A.csv" ("name or relative path") "Camera_Bot_B.csv" ("name or relative path")] -> w434
      frame "Auto Detect", Default {
        n207 = local read "Personality"() -> (w459:string)
        n208 = Equal?(x=w459, y="Sting") -> (x = y?=w461:bool)
        n209 = Select(t="Camera_Bot_A.csv" ("name or relative path"), s=w461, f="Camera_Bot_B.csv" ("name or relative path")) -> (s? t:f=w458:string)
      }
      frame "Sting" {
      }
      frame "Sister-Sting" {
      }
    }
    n210 = Less?(x=w441, y=10) -> (x < y?=w440:bool)
    n211 = Compound Arithmetic op=OR(w440, "Reload", w436) -> (w443:bool)
    n212 = case shown="True" w443 {
      tunnel: w438 -> [_ w556]
      tunnel: w434 -> [_ w548]
      frame False {
      }
      frame True {
        n213 = call "ColorReader.vi"("file path (dialog if empty)"=w556, "name or relative path"="Red.csv") -> ("ColorSettings"=w554:T3)
        n214 = call "ColorReader.vi"("file path (dialog if empty)"=w556, "name or relative path"="Blue.csv") -> ("ColorSettings"=w553:T3)
        n215 = local write "Red Settings"(w554) -> ()
        n216 = local write "Blue Settings"(w553) -> ()
        n217 = call "ColorReader.vi"("file path (dialog if empty)"=w556, "name or relative path"="Purple.csv") -> ("ColorSettings"=w555:T3)
        n218 = call "CameraReader.vi"("file path (dialog if empty)"=w556, "name or relative path"=w548) -> ("User Settings"=w552:T23, "Camera Settings"=w561:T24)
        n219 = local write "Purple Settings"(w555) -> ()
        n220 = Unbundle(w552) -> ("SteadyTime"=w551:dbl, "TargetMarMax"=w550:dbl, "TargetMarMin"=w549:dbl)
        n221 = Unbundle(w561) -> (w573:cluster{"LFOV":dbl, "RFOV":dbl, "CamW":dbl}, w572:cluster{"Ladj":dbl, "Radj":dbl, "Dadj":dbl}, w571:cluster{"CamM":dbl, "CamB":dbl, "AngM":dbl}, "Color"=w557:u16)
        n222 = local write "LED Colors"(w557) -> ()
        n223 = local write "SteadyTimeLimit"(w551) -> ()
        n224 = local write "TargetMarginMax"(w550) -> ()
        n225 = local write "TargetMarginMin"(w549) -> ()
        n226 = Unbundle(w573) -> ("LFOV"=w570:dbl, "RFOV"=w569:dbl, "CamW"=w568:dbl)
        n227 = Unbundle(w572) -> ("Ladj"=w567:dbl, "Radj"=w566:dbl, "Dadj"=w565:dbl)
        n228 = Unbundle(w571) -> ("CamM"=w564:dbl, "CamB"=w563:dbl, "AngM"=w562:dbl)
        n229 = local write "Left FOV"(w570) -> ()
        n230 = local write "Right FOV"(w569) -> ()
        n231 = local write "Camera Width"(w568) -> ()
        n232 = local write "Shift Left Camera Right (Pixels)"(w567) -> ()
        n233 = local write "Shift Right Camera  Right (Pixels)"(w566) -> ()
        n234 = local write "Distance Change"(w565) -> ()
        n235 = local write "Distance M Correction"(w564) -> ()
        n236 = local write "Distance B \nCorrection"(w563) -> ()
        n237 = local write "Angle Correction"(w562) -> ()
        "Cam File" <- w548
      }
    }
    n238 = case shown="\"Test\"" "LED Colors" {
      tunnel: [w574 w575 w576 w578] -> w455
      tunnel: w438 -> [_ _ _ w577]
      frame "Blue", Default {
        n239 = local read "Blue Settings"() -> (w574:T3)
      }
      frame "Red" {
        n240 = local read "Red Settings"() -> (w575:T3)
      }
      frame "Purple" {
        n241 = local read "Purple Settings"() -> (w576:T3)
      }
      frame "Test" {
        n242 = Bundle("Hue"="Hue", "Saturation"="Saturation", "Luminance"="Luminance") -> (w583:T25)  [unwired: 1 in]
        n243 = Bundle("Hue"="Hue", "Sat"="Sat", "Lum"="Lum") -> (w582:cluster{"Hue":i32, "Sat":i32, "Lum":i32})  [unwired: 1 in]
        n244 = Bundle(w583, w582) -> (w578:T26)  [unwired: 1 in]
        n245 = case shown="True" "Write Purple" {
          tunnel: w577 -> [_ w595]
          tunnel: w578 -> [_ w593]
          frame False {
          }
          frame True {
            n246 = call "Writer.vi"("Color Settings"=w593, "FileName"="Purple.csv" ("name or relative path"), "FilePath"=w595) -> ()  [unwired: 9 in]
          }
        }
        n247 = case shown="True" "Write Blue" {
          tunnel: w578 -> [_ w598]
          tunnel: w577 -> [_ w597]
          frame False {
          }
          frame True {
            n248 = call "Writer.vi"("Color Settings"=w598, "FileName"="Blue.csv" ("name or relative path"), "FilePath"=w597) -> ()  [unwired: 9 in]
          }
        }
        n249 = case shown="True" "Write Red" {
          tunnel: w577 -> [_ w592]
          tunnel: w578 -> [_ w590]
          frame False {
          }
          frame True {
            n250 = call "Writer.vi"("Color Settings"=w590, "FileName"="Red.csv" ("name or relative path"), "FilePath"=w592) -> ()  [unwired: 9 in]
          }
        }
      }
    }
    n251 = case shown="True" "Calibrate Cameras" {
      frame False {
      }
      frame True {
        n252 = local read "X1"() -> (w470:dbl)
        n253 = local read "X2"() -> (w471:dbl)
        n254 = flat-sequence {
          tunnel: w470 -> [w489]
          tunnel: w471 -> [w488]
          tunnel: "Distance to Target" -> [w480]
          tunnel: [w486] -> w478
          tunnel: [w485] -> w477
          tunnel: [w484] -> w476
          tunnel: [w483] -> w475
          tunnel: [w482] -> w474
          tunnel: [w481] -> w473
          tunnel: [w480] -> w472
          tunnel: w478 -> [w521]
          tunnel: w477 -> [w520]
          tunnel: w476 -> [w519]
          tunnel: w475 -> [w518]
          tunnel: w474 -> [w516]
          tunnel: w473 -> [w515]
          tunnel: w472 -> [w514]
          tunnel: [w513] -> w467
          tunnel: [w512] -> w466
          tunnel: w469 -> [w511]
          tunnel: w468 -> [w510]
          frame #0 {
            n255 = while {
              tunnel: w489 -> [w494]
              tunnel: w488 -> [w493]
              shift-right: [w495] -> w486
              shift-left: 0.0 ("Distance Change") -> [w496]
              tunnel: [w492] -> w485
              tunnel: [w491] -> w484
              tunnel: [w490] -> w483
              tunnel: [w494] -> w482
              tunnel: [w493] -> w481
              stop <- w499 stop-if-true
              n256 = local read "Camera Width"() -> (w492:dbl)
              n257 = local read "Right FOV"() -> (w491:dbl)
              n258 = local read "Left FOV"() -> (w490:dbl)
              n259 = call "CameraVision.vi"("X2 Change"=w496, "X1 Change"=0.0, "W"=w492, "Distance Change"=0.0, "x2"=w493, "x"=w494, "Left FOV"=w490, "Right FOV"=w491) -> ("Angle to Target"=w498:dbl)  [unwired: 1 in, 1 out]
              n260 = Absolute Value(x=w498) -> (abs(x)=w501:dbl)
              n261 = Greater Than 0?(x=w498) -> (x > 0?=w497:bool)
              n262 = case shown="False" w497 {
                tunnel: w496 -> [w504 w508]
                tunnel: [w505 w509] -> w495
                frame False {
                  n263 = Add(x=w504, y=0.1) -> (x+y=w505:dbl)
                }
                frame True {
                  n264 = Subtract(x=w508, y=0.1) -> (x-y=w509:dbl)
                }
              }
              n265 = Less?(x=w501, y=0.01) -> (x < y?=w499:bool)
            }
          }
          frame #1 {
            n266 = while {
              tunnel: w521 -> [w527]
              tunnel: w520 -> [w537]
              tunnel: w519 -> [w536]
              tunnel: w518 -> [w535]
              shift-right: [w531] -> w512
              shift-left: 0.0 ("Distance Change") -> [w532]
              tunnel: w516 -> [w534]
              tunnel: w515 -> [w533]
              tunnel: w514 -> [w530]
              tunnel: [w527] -> w513
              tunnel: w511 -> [w523]
              tunnel: w510 -> [w522]
              stop <- w538 stop-if-true
              n267 = call "CameraVision.vi"("X2 Change"=w527, "X1 Change"=0.0, "W"=w537, "Distance Change"=w532, "x2"=w533, "x"=w534, "Left FOV"=w535, "Right FOV"=w536) -> ("Distance to Target"=w526:dbl)  [unwired: 1 in, 1 out]
              n268 = Multiply(x=w526, y=w523) -> (x*y=w525:dbl)
              n269 = Add(x=w525, y=w522) -> (x+y=w524:dbl)
              n270 = Subtract(x=w530, y=w524) -> (x-y=w529:dbl)
              n271 = Absolute Value(x=w529) -> (abs(x)=w540:dbl)
              n272 = Greater Than 0?(x=w529) -> (x > 0?=w528:bool)
              n273 = case shown="False" w528 {
                tunnel: w532 -> [w544 w547]
                tunnel: [w542 w545] -> w531
                frame False {
                  n274 = Add(x=w544, y=0.005) -> (x+y=w542:dbl)
                }
                frame True {
                  n275 = Subtract(x=w547, y=0.1) -> (x-y=w545:dbl)
                }
              }
              n276 = Less?(x=w540, y=0.01) -> (x < y?=w538:bool)
            }
          }
        }
        n277 = local read "Distance M Correction"() -> (w469:dbl)
        n278 = local read "Distance B \nCorrection"() -> (w468:dbl)
        n279 = local write "Shift Right Camera  Right (Pixels)"(w467) -> ()
        n280 = local write "Distance Change"(w466) -> ()
      }
    }
    n281 = Cluster To Array(cluster="Score Lower Limits") -> (array=→"ScoreLowerLimitsA":dbl[])
    n282 = Unbundle(w455) -> (w453:T25, w454:cluster{"Hue":i32, "Sat":i32, "Lum":i32})
    n283 = Unbundle(w453) -> ("Hue"=w450:i32, "Saturation"=w451:i32, "Luminance"=w452:i32)
    n284 = call "Compute HSL Color Ranges.vi"("Margins"=w454, "Luminance"=w452, "Saturation"=w451, "Hue"=w450) -> ("Lum Range"=→"Lum Range":cluster{i32, i32}, "Sat Range"=→"Sat Range":cluster{i32, i32}, "Hue Range"=→"Hue Range":cluster{i32, i32})  [unwired: 5 in]
  }
  n285 = Build Path(base path=w92, name or relative path=w90) -> (appended path=w81:path)
  n286 = call <vilib>:"WPI_CameraSet White Balance.vi"("error in (no error)"=w54, "White Balance"="White Balance", "CameraDevRef"=w55) -> ("error out"=w74:errorcluster, "CameraDevRef Out"=w75:T21)  [unwired: 7 out]
  n287 = call <vilib>:"WPI_CameraSet White Balance.vi"("error in (no error)"=w52, "White Balance"="White Balance", "CameraDevRef"=w53) -> ("error out"=w79:errorcluster, "CameraDevRef Out"=w80:T21)  [unwired: 7 out]
  n288 = while {
    tunnel: w81 -> [w600]
    stop <- FALSE stop-if-true
    # "The Write To Spreadsheet File.vi opens,\n writes to, and closes the specified file."
    n289 = while {
      shift-right: [w638] -> w602
      shift-left: string[] [] -> [w637]
      i -> [w633]
      stop <- w635 stop-if-true
      w612 = "," ("delimiter (Tab)")
      n290 = Wait (ms)(milliseconds to wait=u32 100) -> ()  [unwired: 1 out]
      n291 = local read "Collector System Enabled"() -> (w622:bool)
      n292 = local read "Turret Postition"() -> (w630:cluster{dbl, dbl})
      n293 = local read "TargetAcquired"() -> (w617:bool)
      n294 = local read "Shooter RPM"() -> (w631:cluster{dbl, dbl})
      n295 = local read "Distance From Target"() -> (w627:dbl)
      n296 = local read "FIRE!"() -> (w618:bool)
      n297 = local read "Angle to Target"() -> (w628:dbl)
      n298 = local read "Battery Voltage"() -> (w629:dbl)
      n299 = Unbundle(w630) -> (w623:dbl)  [unwired: 1 out]
      n300 = Unbundle(w631) -> (w626:dbl)  [unwired: 1 out]
      n301 = Boolean To (0,1)(Boolean=w622) -> (0, 1=w621:i16)
      n302 = Boolean To (0,1)(Boolean=w618) -> (0, 1=w620:i16)
      n303 = Boolean To (0,1)(Boolean=w617) -> (0, 1=w619:i16)
      n304 = local read "compass lag"() -> (w606:dbl)
      n305 = local read "Status"() -> (w615:T1)
      n306 = local read "Mode"() -> (w616:enum8{"Tele-Op", "Auto", ""})
      n307 = local read "Gyro"() -> (w624:dbl)
      n308 = local read "FPS"() -> (w625:dbl)
      n309 = local read "Compass"() -> (w607:dbl)
      n310 = Insert Into Array(array=dbl[] [], new element #1=w629, new element #2=w628, new element #3=w627, new element #4=w626, new element #5=w625, new element #6=w624, new element #7=w623, new element #8=w621, new element #9=w620, new element #10=w619, new element #11=w616, new element #12=w615, new element #13=w607, new element #14=w606) -> (w632:dbl[])  [unwired: 1 in]
      n311 = Array To Spreadsheet String(delimiter (Tab)=w612, array=w632, 3:"%.2f" ("format string")) -> (spreadsheet string=w610:string)
      n312 = Get Date/Time In Seconds() -> (seconds since 1Jan1904=w639:timestamp)
      n313 = Search/Split String(string=w610, search string/char (-)="\r\n") -> (substring before match=w609:string)  [unwired: 1 in, 2 out]
      n314 = Get Date/Time String(seconds (now)=w639, want seconds? (F)=TRUE) -> (time string=w613:string)  [unwired: 1 in, 1 out]
      n315 = Concatenate Strings(w613, w612, w609, w612) -> (w608:string)
      n316 = Greater Or Equal?(x=w633, y=10) -> (x >= y?=w635:bool)
      n317 = Insert Into Array(array=w637, index=w633, new element=w608) -> (w638:string[])
    }
    n318 = call-poly <vilib>:"Write To Spreadsheet File.vi"("delimiter (\\t)"="," ("delimiter (\\t)"), "transpose? (no:F)"=TRUE, "append to file? (new file:F)"=TRUE, "1D data"=w602, "file path (dialog if empty)"=w600) -> ()  [unwired: 3 in, 1 out]
  }
  n319 = call <vilib>:"WPI_CameraSet Exposure.vi"("error in (no error)"=w74, "Exposure"="Exposure", "CameraDevRef"=w75) -> ("error out"=w59:errorcluster, "CameraDevRef Out"=w58:T21)  [unwired: 7 out]
  n320 = call <vilib>:"WPI_CameraSet Exposure.vi"("error in (no error)"=w79, "Exposure"="Exposure", "CameraDevRef"=w80) -> ("error out"=w57:errorcluster, "CameraDevRef Out"=w56:T21)  [unwired: 7 out]
  n321 = call <vilib>:"WPI_CameraSet Brightness.vi"("error in (no error)"=w59, "Brightness"="Brightness", "CameraDevRef"=w58) -> ("error out"=w71:errorcluster, "CameraDevRef Out"=w72:T21)  [unwired: 7 out]
  n322 = call <vilib>:"WPI_CameraSet Brightness.vi"("error in (no error)"=w57, "Brightness"="Brightness", "CameraDevRef"=w56) -> ("error out"=w76:errorcluster, "CameraDevRef Out"=w33:T21)  [unwired: 7 out]
  n323 = call <vilib>:"WPI_CameraAcquire MJPG Loop.vi"("CameraDevRef"=w72) -> ()  [unwired: 11 in]
  n324 = call <vilib>:"WPI_CameraAcquire MJPG Loop.vi"("CameraDevRef"=w33) -> ()  [unwired: 11 in]
  n325 = call <vilib>:"WPI_CameraStart.vi"("error in (no error)"=w71, "CameraDevRef"=w72) -> ("error out"=w23:errorcluster, "CameraDevRef Out"=w18:T21)  [unwired: 8 in]
  n326 = call "IMAQ Create"("Image Name"="Mask", "Image Type"=w9) -> ("New Image"=w8:T2)  [unwired: 2 in, 2 out]
  n327 = call "IMAQ Create"("Image Name"="Orig", "Image Type"=w7) -> ("New Image"=w5:T2)  [unwired: 2 in, 2 out]
  n328 = call "IMAQ Create"("Image Name"="Raw Orig", "Image Type"=w30) -> ("New Image"=w25:T2)  [unwired: 2 in, 2 out]
  n329 = call "IMAQ Create"("Image Name"="Mask2", "Image Type"=w12) -> ("New Image"=w11:T2)  [unwired: 2 in, 2 out]
  n330 = call "IMAQ Create"("Image Name"="Orig2", "Image Type"=w16) -> ("New Image"=w14:T2)  [unwired: 2 in, 2 out]
  n331 = call "IMAQ Create"("Image Name"="Raw Orig 2", "Image Type"=w28) -> ("New Image"=w27:T2)  [unwired: 2 in, 2 out]
  n332 = call <vilib>:"WPI_CameraStart.vi"("error in (no error)"=w76, "CameraDevRef"=w33) -> ("error out"=w20:errorcluster, "CameraDevRef Out"=w17:T21)  [unwired: 8 in]
  n333 = call <vilib>:"Simple Error Handler.vi"("type of dialog (OK msg:1)"=w22, "error in (no error)"=w23) -> ()  [unwired: 3 in, 5 out]
  n334 = call <vilib>:"Simple Error Handler.vi"("type of dialog (OK msg:1)"=w21, "error in (no error)"=w20) -> ()  [unwired: 3 in, 5 out]
  n335 = while {
    tunnel: w25 -> [w678]
    tunnel: "Camera Settings" -> [w677]
    tunnel: w17 -> [w674]
    tunnel: w8 -> [w652]
    tunnel: w5 -> [w656]
    tunnel: "Private CHull Dest" ("Image Name") -> [w644]
    i -> [w654]
    stop <- FALSE stop-if-true
    w642 = u16 1 items=["RGB", "HSL", "HSV", "HSI"] ("Color Mode")
    w662 = T17 0 items=["no dialog", "OK message", "continue or stop message", "OK message + warnings", "continue/stop + warnings"] ("type of dialog (OK msg:1)")
    w676 = "10.8.36.12"  # Left Camera Address
    # "Sub Frame is the number of the fram processed.  Used by other tasks for synchronization and throttling."
    # "This Loop processes the images from the Right Camera and gives the highest rectangle found that\npasses the rectangle filters."
    n336 = call <vilib>:"WPI_CameraUpdate Camera Status.vi"("CameraDevRef In"=w674, "Enable Vision"=TRUE) -> ()  [unwired: 3 in, 1 out]
    n337 = call <vilib>:"WPI_CameraRead MJPG.vi"("Operation"=enum16{"Read", "Reopen", "Close"}."Read", "Camera Settings"=w677, "Image"=w678, "address"=w676) -> ("error out"=w655:errorcluster, "Image Out"=w645:T2)  [unwired: 5 in, 1 out]
    "Raw Image Out" <- w645
    n338 = call "IMAQ Copy"("error in (no error)"=w655, "Image Dst"=w656, "Image Src"=w645) -> ("error out"=w665:errorcluster, "Image Dst Out"=w666:T2)  [unwired: 3 in]
    n339 = local read "Lum Range"() -> (w647:cluster{i32, i32})
    n340 = local read "Hue Range"() -> (w648:cluster{i32, i32})
    n341 = local read "Sat Range"() -> (w646:cluster{i32, i32})
    n342 = call "IMAQ Extract"("Optional Rectangle"=i32[] [400, 0, 640, 480], "error in (no error)"=w665, "Image Src"=w666) -> ("error out"=w651:errorcluster, "Image Dst Out"=w653:T2)  [unwired: 7 in]
    n343 = local read "Particle Count Limit"() -> (w667:i32)
    n344 = local read "Area Size Limit"() -> (w668:i32)
    n345 = call "IMAQ ColorThreshold"("Blue or Luma or Val or Inten Range"=w647, "Green or Sat Range"=w646, "Color Mode"=w642, "error in (no error)"=w651, "Red or Hue Range"=w648, "Image Dst"=w652, "Image Src"=w653) -> ("error out"=w649:errorcluster, "Image Dst Out"=w650:T2)  [unwired: 3 in]
    n346 = local read "Aspect Ratio Upper"() -> (w670:dbl)
    n347 = local read "ScoreLowerLimitsA"() -> (w669:dbl[])
    n348 = call "Score Particles.vi"("error in (no error)"=w649, "Area Size Limit"=w668, "Particle Count Limit"=w667, "Image Name"=w644, "Image Refnum in"=w650) -> ("error out"=w664:errorcluster, "Scored Particle Info"=w660:T4, "Image Refnum out"=→"Processed Image Source":T2)  [unwired: 4 in]
    "Scored Particle Info" <- w660
    n349 = call <vilib>:"Simple Error Handler.vi"("type of dialog (OK msg:1)"=w662, "error in (no error)"=w664) -> ()  [unwired: 3 in, 5 out]
    n350 = Array Size(array=w660) -> (size(s)=w658:i32)
    n351 = Greater Than 0?(x=w658) -> (x > 0?=w659:bool)
    n352 = for {
      N: w658 -> [_]
      tunnel: w660 -> [w692]
      tunnel: [w691] -> w657
      tunnel: w669 -> [w690]
      tunnel: w670 -> [w689]
      i -> [w693]
      n353 = call "Rectangle Filter.vi"("Aspect Ratio Upper"=w689, "Index Value"=w693, "Lower Limits"=w690, "Scored Particle Info"=w692, "Left"=TRUE) -> ("Index of Top Rectangle"=w691:i32)  [unwired: 1 in]
    }
    n354 = in-place {
      in-place-border: [w685] -> w672
      in-place-border: w660 -> [w687]
      in-place-border: w657 -> [w686]
      in-place-border: [w684] -> w671
      in-place-border: w659 -> [w683]
      in-place-border: [w682] -> w673
      in-place-border: [w681] -> w663
      n355 = call "Mask Calculations.vi"("Any Targets"=w683, "Index of Top Rectangle"=w686, "Scored Particle Info"=w687) -> ("Vertical Center of Rectangle"=w682:dbl, "Valid Target"=w684:bool, "Horizontal Center of Rectangle"=w685:dbl, "Cluster"=w681:T5)  [unwired: 5 in]
    }
    "Left Target" <- w663
    "Left Target Valid" <- w671
    "X1" <- w672
    "Y1" <- w673
    "SubFrame1" <- w654
  }
  n356 = while {
    tunnel: w18 -> [w732]
    tunnel: w27 -> [w731]
    tunnel: "Camera Settings" -> [w729]
    tunnel: w14 -> [w713]
    tunnel: w11 -> [w707]
    tunnel: "Private CHull Dest 2" ("Image Name") -> [w696]
    i -> [w710]
    stop <- FALSE stop-if-true
    w694 = u16 1 items=["RGB", "HSL", "HSV", "HSI"] ("Color Mode")
    w719 = T17 0 items=["no dialog", "OK message", "continue or stop message", "OK message + warnings", "continue/stop + warnings"] ("type of dialog (OK msg:1)")
    w730 = "10.8.36.11"  # Right Camera Address
    n357 = call <vilib>:"WPI_CameraUpdate Camera Status.vi"("CameraDevRef In"=w732, "Enable Vision"=TRUE) -> ()  [unwired: 3 in, 1 out]
    n358 = call <vilib>:"WPI_CameraRead MJPG.vi"("Operation"=enum16{"Read", "Reopen", "Close"}."Read", "Camera Settings"=w729, "Image"=w731, "address"=w730) -> ("error out"=w711:errorcluster, "Image Out"=w712:T2)  [unwired: 5 in, 1 out]
    "Raw Image Out 2" <- w712
    n359 = call "IMAQ Copy"("error in (no error)"=w711, "Image Dst"=w713, "Image Src"=w712) -> ("error out"=w721:errorcluster, "Image Dst Out"=w722:T2)  [unwired: 3 in]
    n360 = local read "Lum Range"() -> (w704:cluster{i32, i32})
    n361 = local read "Hue Range"() -> (w706:cluster{i32, i32})
    n362 = local read "Sat Range"() -> (w705:cluster{i32, i32})
    n363 = call "IMAQ Extract"("Optional Rectangle"=i32[] [0, 0, 240, 480] ("Optional Rectangle 2"), "error in (no error)"=w721, "Image Src"=w722) -> ("error out"=w709:errorcluster, "Image Dst Out"=w708:T2)  [unwired: 7 in]
    n364 = local read "Particle Count Limit"() -> (w702:i32)
    n365 = local read "Area Size Limit"() -> (w701:i32)
    n366 = call "IMAQ ColorThreshold"("Blue or Luma or Val or Inten Range"=w704, "Green or Sat Range"=w705, "Color Mode"=w694, "error in (no error)"=w709, "Red or Hue Range"=w706, "Image Dst"=w707, "Image Src"=w708) -> ("error out"=w700:errorcluster, "Image Dst Out"=w703:T2)  [unwired: 3 in]
    n367 = local read "Aspect Ratio Upper"() -> (w724:dbl)
    n368 = local read "ScoreLowerLimitsA"() -> (w723:dbl[])
    n369 = call "Score Particles.vi"("error in (no error)"=w700, "Area Size Limit"=w701, "Particle Count Limit"=w702, "Image Name"=w696, "Image Refnum in"=w703) -> ("error out"=w697:errorcluster, "Scored Particle Info"=w698:T4, "Image Refnum out"=→"Processed Image 2 Source":T2)  [unwired: 4 in]
    "Scored Particle Info 2" <- w698
    n370 = call <vilib>:"Simple Error Handler.vi"("type of dialog (OK msg:1)"=w719, "error in (no error)"=w697) -> ()  [unwired: 3 in, 5 out]
    n371 = Array Size(array=w698) -> (size(s)=w717:i32)
    n372 = Greater Than 0?(x=w717) -> (x > 0?=w718:bool)
    n373 = for {
      N: w717 -> [_]
      tunnel: w698 -> [w746]
      tunnel: [w745] -> w716
      tunnel: w723 -> [w744]
      tunnel: w724 -> [w743]
      i -> [w747]
      n374 = call "Rectangle Filter.vi"("Aspect Ratio Upper"=w743, "Index Value"=w747, "Lower Limits"=w744, "Scored Particle Info"=w746, "Left"=FALSE) -> ("Index of Top Rectangle"=w745:i32)  [unwired: 1 in]
    }
    n375 = in-place {
      in-place-border: [w739] -> w715
      in-place-border: w698 -> [w741]
      in-place-border: w716 -> [w740]
      in-place-border: [w738] -> w726
      in-place-border: w718 -> [w737]
      in-place-border: [w736] -> w727
      in-place-border: [w735] -> w720
      n376 = call "Mask Calculations.vi"("Any Targets"=w737, "Index of Top Rectangle"=w740, "Scored Particle Info"=w741) -> ("Vertical Center of Rectangle"=w736:dbl, "Valid Target"=w738:bool, "Horizontal Center of Rectangle"=w739:dbl, "Cluster"=w735:T5)  [unwired: 5 in]
    }
    "Right Target" <- w720
    "Right Target Valid" <- w726
    "Y2" <- w727
    n377 = Subtract(x=480.0, y=w715) -> (x-y=→"X2":dbl)
    "SubFrame2" <- w710
  }
  n378 = call-poly <vilib>:"Write To Spreadsheet File.vi"("delimiter (\\t)"="," ("delimiter (\\t)"), "format (%s)"="%s", "1D data"=string[] ["Time", "Batt(Volts)", "Ang_To_Tar(Deg)", "Dist_To_Tar(Feet)", "Shooter_RPM(RMP)", "FPS(Frame per second)", "Gyro(Degrees)", "Turret Postion (Degree)", "Collector System Enabled (TRUE/FALSE)", "FIRE (TRUE/FALSE)", "Target Acquired (TRUE/FALSE)", "Mode", "Status", "J1B1", "J1B2", "J1B3", "J1B4", "J1B5", "J1B6", "J1B7", "J1B8", "J2B1", "J2B2", "J2B3", "J2B4", "J2B5", "J2B6", "J2B7", "J2B8"], "file path (dialog if empty)"=w81) -> ()  [unwired: 4 in, 1 out]
